vi "HISTO_READ_COUNT.vi"(0 "TCP Network Connection in":refnum<k5>, 5 "error in (no error)":errorcluster) -> (14 "TCP Network Connection out":refnum<k5>, 16 "VALUE":u32, 17 "STATUS":u32, 19 "error out":errorcluster)   [LabVIEW 2019, in "Histogram.lvlib"]
uses:
  Histogram.lvlib
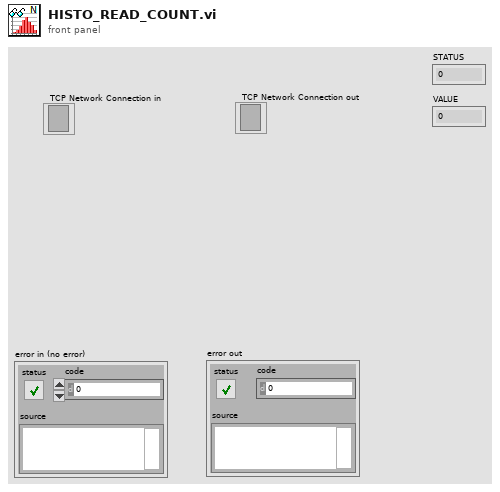
[diagram p1: front panel]
types:
  T1 = enum16{"big-endian, network order", "native, host order", "little-endian"}
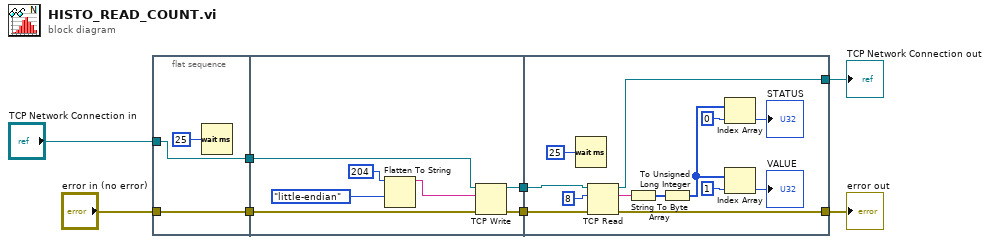
[diagram p0: block diagram]
diagram:
  n1 = flat-sequence {
    tunnel: [w10] -> w4
    tunnel: [w11] -> w3
    tunnel: "error in (no error)" -> [w11]
    tunnel: "TCP Network Connection in" -> [w10]
    tunnel: w4 -> [w18]
    tunnel: w3 -> [w17]
    tunnel: [w16] -> w2
    tunnel: [w15] -> w1
    tunnel: [w28] -> w6
    tunnel: [w29] -> w5
    tunnel: w2 -> [w31]
    tunnel: w1 -> [w30]
    frame #0 {
      n2 = Wait (ms)(milliseconds to wait=u32 25) -> ()  [unwired: 1 out]
    }
    frame #1 {
      n3 = Flatten To String(anything=u32 204 ("element"), byte order (0:big-endian, network order)=T1."little-endian") -> (data string=w12:string)  [unwired: 2 in, 2 out]
      n4 = TCP Write(connection ID=w18, data in=w12, error in (no error)=w17) -> (connection ID out=w16:refnum<k5>, error out=w15:errorcluster)  [unwired: 1 in, 1 out]
    }
    frame #2 {
      n5 = Wait (ms)(milliseconds to wait=u32 25) -> ()  [unwired: 1 out]
      n6 = TCP Read(connection ID=w31, bytes to read=8, error in (no error)=w30) -> (connection ID out=w29:refnum<k5>, data out=w25:string, error out=w28:errorcluster)  [unwired: 2 in]
      n7 = String To Byte Array(string=w25) -> (unsigned byte array=w24:u8[])
      n8 = To Unsigned Long Integer(number=w24) -> (unsigned 32bit integer=w23:u32[])
      n9 = Index Array(array=w23, index=0) -> (element=→"STATUS":u32)
      n10 = Index Array(array=w23, index=1) -> (element=→"VALUE":u32)
    }
  }
  "error out" <- w6
  "TCP Network Connection out" <- w5
